vi "PH_Sixpack.PC SetStopSwitchLimits.vi"(0 "i ref in":refnum<vi>, 1 "axis":i32=-1, 2 "Stopswitch Limits":T1={"MinLeft(0)"=150, "MaxRight(1023)"=900}, 3 "To set?":bool, 5 "error in":errorcluster) -> (14 "i ref out":refnum<vi>, 16 "ok?":bool, 19 "error out":errorcluster)   [LabVIEW 2014, in "PH_Sixpack.lvlib"]
doc: "This VI stores information to own attributes."
uses:
  PH_Sixpack.lvlib
  instr.lib/Sixpack/PackDLL/Stopswitch Limits.ctl
  instr.lib/Sixpack/Sixpack - Driver.lvlib
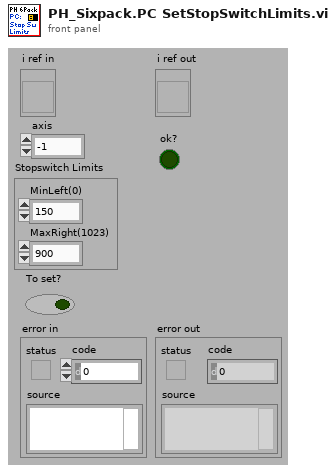
[diagram p1: front panel]
types:
  T1 = typedef "Sixpack - Driver.lvlib/Stopswitch Limits.ctl" = cluster{"MinLeft(0)":u16, "MaxRight(1023)":u16}
  T2 = typedef "PH_Sixpack.lvlib/PH_Sixpack.i attribute.ctl" = cluster{"Information":cluster{"SixPack ID(0)":u16, "BaudRate(19200)":u16, "COM Port":enum32{"COM1", "COM2", "COM3", "COM4", "COM5", "COM6", "COM7", "COM8", "COM9"}, "HANDLE":i32}, "Serial Number":dbl, "Firmwareversion":dbl, "Axes":T3[], "Status":T14, "Axis to do a RefSearch":i32, "GUI Refs":cluster{"Information":refnum<vi>, "Serial Number":refnum<vi>, "Firmwareversion":refnum<vi>, "Status":refnum<vi>, "Axis to do a RefSearch":refnum<vi>, "Axes Configuration (Sixpack)":refnum<vi>, "Inputs":refnum<vi>, "PeriodicInterval [ms]":refnum<vi>}, "Constructor finished":bool, "Ignore Error":bool}
  T3 = typedef "PH_Sixpack.lvlib/PH_Sixpack.Axis Cluster.ctl" = cluster{"Config":T4, "To set?":cluster{"VmaxAmax":bool, "I max":bool, "VStartVminDivi":bool, "Ref Search Parameter":bool, "Stopswitch Limits":bool, "Axis Parameter":bool, "I Control":bool}}
  T4 = typedef "PH_Sixpack.lvlib/PH_Sixpack.Axis Configuration.ctl" = cluster{"VmaxAmax":T5, "I max (50%)":T6, "VStartVminDivi":T7, "Ref Search Parameter":T8, "Stopswitch Limits":T1, "Axis Parameter":T9, "I Control":T12}
  T5 = typedef "Sixpack - Driver.lvlib/VmaxAmax.ctl" = cluster{"VMax(511)":u16, "AMax(128)":u16}
  T6 = typedef "Sixpack - Driver.lvlib/PeakCurrent.ctl" = dbl
  T7 = typedef "Sixpack - Driver.lvlib/VStartVmin.ctl" = cluster{"VStart(5)":u16, "Vmin(4)":u16, "Div i (2)":enum8{"0", "1", "2", "3"}}
  T8 = typedef "Sixpack - Driver.lvlib/Ref Search Parameter.ctl" = cluster{"VRefMax(100)":u16, "DebouncingTime (22ms)":u8}
  T9 = typedef "Sixpack - Driver.lvlib/Motor Parameter.ctl" = cluster{"Poslimit (6400)":u32, "P5 Bits":T10, "P6 Bits":T11}
  T10 = typedef "Sixpack - Driver.lvlib/MotorParameter_P5.ctl" = cluster{"MT_PI":bool, "MT_ROTARY":bool, "MT_AUTONULLCMD":bool, "MT_TESTNULL":bool, "MT_NULLLEFT":bool, "MT_NULLCENTRE":bool, "MT_STOPNULL":bool, "MT_FILTERSWITCH":bool}
  T11 = typedef "Sixpack - Driver.lvlib/MotorParameter_P6.ctl" = cluster{"MT_OPTIMIZEWAY":bool, "MT_FASTREF":bool, "MT_MECHREF":bool, "MT_DELAYTESTNULL":bool, "MT_STOPSOFT":bool, "MT_STOPNOREF":bool, "MT_NULLPOSITIVE":bool, "MUT_STOPFULSTEPS":bool}
  T12 = typedef "Sixpack - Driver.lvlib/Current Control.ctl" = cluster{"PowerDownDelay (500)":u16, "PowerDown (0%)":T13, "Standing (50%)":T13, "Running (75%)":T13, "Accelerating (100%)":T13}
  T13 = typedef "Sixpack - Driver.lvlib/Current.ctl" = enum8{"100%", "75%", "50%", "38%", "25%", "19%", "13%", "9%", "0%"}
  T14 = typedef "PH_Sixpack.lvlib/PH_Sixpack.Status.ctl" = enum32{"None", "Init", "Configure", "configured", "Close", "closed"}
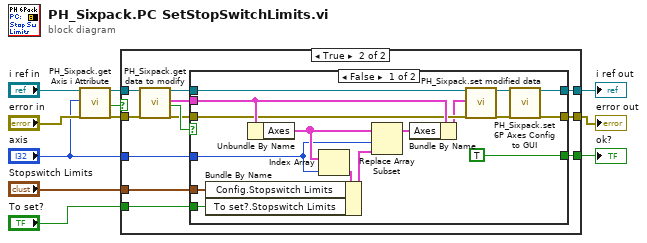
[diagram p0: block diagram]
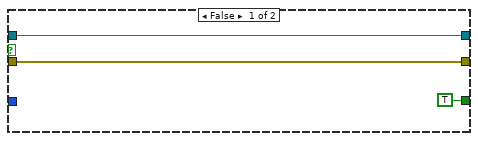
[diagram p2: hidden frame]
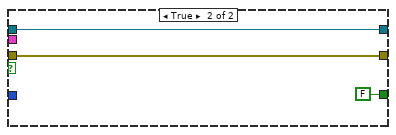
[diagram p3: hidden frame]
diagram:
  n1 = call "PH_Sixpack.get Axis i Attribute.vi"("VI in"="i ref in", "Axis"="axis", "error in"="error in") -> ("VI out"=w6:refnum<vi>, "Axis found?"=w3:bool, "error out"=w8:errorcluster)  [unwired: 10 in, 4 out]
  n2 = case shown="True" w3 {
    tunnel: w6 -> [w14 w26]
    tunnel: w8 -> [w13 w25]
    tunnel: [w13 w22] -> w10
    tunnel: [w14 w20] -> w9
    tunnel: "axis" -> [_ w18]
    tunnel: "Stopswitch Limits" -> [_ w17]
    tunnel: "To set?" -> [_ w16]
    tunnel: [TRUE w15] -> w1
    frame False {
    }
    frame True {
      n3 = call "PH_Sixpack.get data to modify.vi"("i ref in"=w26, "error in (no error)"=w25) -> ("i ref out"=w21:refnum<vi>, "i attribute"=w19:T2, "timed out"=w24:bool, "error out"=w23:errorcluster)  [unwired: 14 in]
      n4 = case shown="False" w24 {
        tunnel: [w29 w45] -> w22
        tunnel: w23 -> [w37 w45]
        tunnel: [w27 w44] -> w20
        tunnel: w21 -> [w38 w44]
        tunnel: w19 -> [w41 _]
        tunnel: w18 -> [w35 _]
        tunnel: w17 -> [w32 _]
        tunnel: w16 -> [w31 _]
        tunnel: [TRUE FALSE] -> w15
        frame False {
          n5 = Unbundle By Name(w41) -> ("Axes"=w40:T3[])
          n6 = Index Array(array=w40, index=w35) -> (element=w39:T3)
          n7 = Bundle By Name(cluster=w39, "Config.Stopswitch Limits"=w32, "To set?.Stopswitch Limits"=w31) -> (w33:T3)
          n8 = Replace Array Subset(array=w40, new element=w33, index=w35) -> (w34:T3[])
          n9 = Bundle By Name(cluster=w41, "Axes"=w34) -> (w36:T2)
          n10 = call "PH_Sixpack.set modified data.vi"("i ref in"=w38, "i attribute"=w36, "error in (no error)"=w37) -> ("i ref out"=w28:refnum<vi>, "error out"=w42:errorcluster)  [unwired: 15 in]
          n11 = call "PH_Sixpack.set 6P Axes Config to GUI.vi"("VI in"=w28, "error in (no error)"=w42) -> ("VI out"=w27:refnum<vi>, "error out"=w29:errorcluster)  [unwired: 16 in]
        }
        frame True {
        }
      }
    }
  }
  "error out" <- w10
  "i ref out" <- w9
  "ok?" <- w1
